vi "sendStop.vi"(8 "error in (no error)":errorcluster, 11 "PixelflySA in":refnum<class "PixelflySA.lvclass">) -> (0 "error out":errorcluster, 3 "PixelflySA out":refnum<class "PixelflySA.lvclass">)   [LabVIEW 2011, in "PixelflySA.lvclass"]
uses:
  PixelflySA.lvclass
  PixelflySA.lvclass/PixelflySA.ctl
  Tools/Filing/FileSystem/FileSystem.lvclass
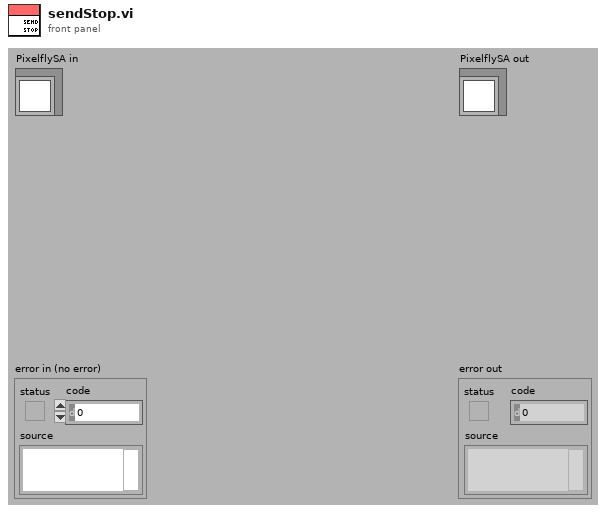
[diagram p1: front panel]
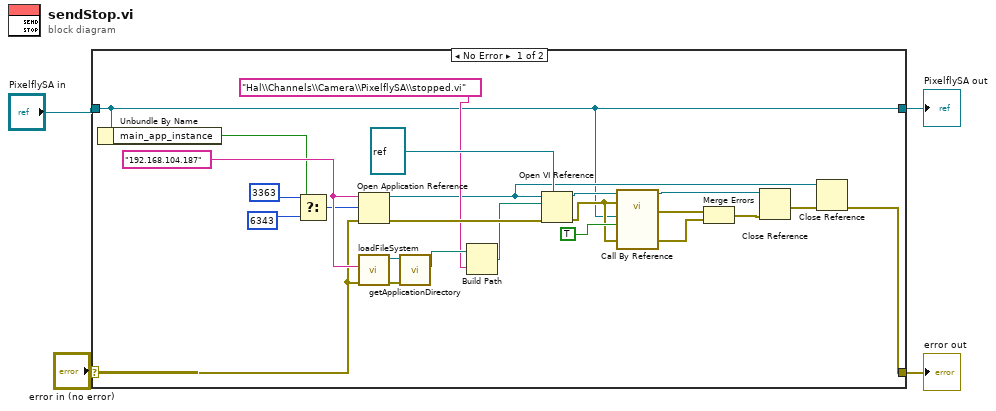
[diagram p0: block diagram]
diagram:
  n1 = case shown="No Error" "error in (no error)" {
    selector: "error in (no error)" -> [w24 w30]
    tunnel: [w11 w30] -> w3
    tunnel: [w9 w29] -> w1
    tunnel: "PixelflySA in" -> [w9 w29]
    frame No Error {
      w25 = "192.168.104.187" ("machine name (\"\":  open local reference)")
      n2 = Unbundle By Name(w9) -> ("main_app_instance"=w8:bool)
      n3 = Select(t=u16 3363 ("port number or service name (3363)"), s=w8, f=u16 6343 ("port number or service name (3363)")) -> (s? t:f=w5:u16)
      n4 = Open Application Reference(8:w24, 10:w5, 11:w25) -> (0:w28:errorcluster, 3:w13:refnum<vi>)  [unwired: 1 in]
      n5 = call "loadFileSystem.vi"("error in (no error)"=w24, "computer name"=w25) -> ("error out"=w26:errorcluster, "FileSystem out"=w10:refnum<class "FileSystem.lvclass">)  [unwired: 8 in]
      n6 = call-dynamic "getApplicationDirectory.vi"("error in (no error)"=w26, "FileSystem.lvclass in"=w10) -> ("ApplicationDirectory"=w23:path)  [unwired: 7 in, 2 out]
      n7 = Build Path(base path=w23, name or relative path="Hal\\Channels\\Camera\\PixelflySA\\stopped.vi" ("viPath")) -> (appended path=w21:path)
      n8 = Open VI Reference(type specifier VI Refnum (for type only)=refnum<vi> refnum, application reference (local)=w13, vi path=w21, error in (no error)=w28) -> (vi reference=w20:refnum<vi>, error out=w18:errorcluster)  [unwired: 2 in]
      n9 = call-by-ref "?"(reference=w20, error in=w18, 8:"error in (no error)"=w18, "stopped"=TRUE, "PixelflySA in"=w9) -> (reference out=w15:refnum<vi>, error out=w17:errorcluster, 0:"error out"=w16:errorcluster)  [unwired: 7 in, 1 out]
      n10 = Merge Errors(w17, w16) -> (w14:errorcluster)
      n11 = Close Reference(reference=w15, error in (no error)=w14) -> (error out=w12:errorcluster)
      n12 = Close Reference(reference=w13, error in (no error)=w12) -> (error out=w11:errorcluster)
    }
    frame Error {
    }
  }
  "error out" <- w3
  "PixelflySA out" <- w1
